vi "PH_Sound.ProcCases.vi"(0 "i ref in":refnum<vi>, 1 "selector":string, 2 "Data":T1, 3 "call cluster":T2={"Object"="", "Selector"="", "CallType"=enum."synchronous", "Async Object"="", "Async Selector"="", "Data Descriptor"="", "Data"=[], "Error #"=0, "Expire"=0}, 5 "error in (no error)":errorcluster) -> (14 "i ref out":refnum<vi>, 17 "answer cluster":T2={"Object"="", "Selector"="", "CallType"=enum."synchronous", "Async Object"="", "Async Selector"="", "Data Descriptor"="", "Data"=[], "Error #"=0, "Expire"=0}, 19 "error out":errorcluster)   [LabVIEW 2014, in "PH_Sound.lvlib"]
doc: "This method is called by a process from within the default case in the event loop. The methods of a class that are linked to events will be called from THIS method. Add your code here."
uses:
  PH_Sound.lvlib
  CS_Core/CSSystem/CoreDefs/CoreDefs.call_type.ctl
  CS_Core/BaseProcess/BaseProcess.descriptor string definition.ctl
  CS_Core/CSSystem/CoreDefs/CoreDefs.rawDataType.ctl
  CS_Core/CSSystem/CoreLib/CoreLib.byte array 2 double.vi
  CS_Core/CSSystem/CoreLib/CoreLib.byte array 2 int.vi
  CS_Core/CSSystem/CoreLib/CoreLib.string 2 byte array.vi
  CS_Core/CSSystem/CoreLib/CoreLib.byte array 2 short.vi
  CS_Core/BaseProcess/BaseProcess.lvlib
  CS_Core/CSSystem/CoreLib/CoreLib.lvlib
  CS_Core/CAEObj/CAEObj.lvlib
  PH_Basics/PH_Common/PH_Common.lvlib
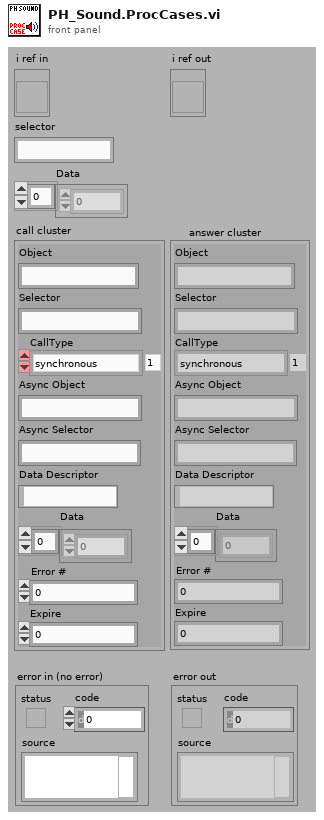
[diagram p1: front panel]
types:
  T1 = typedef "CoreDefs.rawDataType.ctl" = i8[]
  T2 = typedef "CoreDefs.call_type.ctl" = cluster{"Object":string, "Selector":string, "CallType":enum16{"simple", "synchronous", "asynchronous"}, "Async Object":string, "Async Selector":string, "Data Descriptor":T3, "Data":T1, "Error #":i32, "Expire":u32}
  T3 = typedef "BaseProcess.lvlib/BaseProcess.descriptor string definition.ctl" = string
  T4 = typedef "PH_Sound.lvlib/PH_Sound.i attribute.ctl" = cluster{"GUI Refs":cluster{"Exit":refnum<vi>, "Laserfreigabe":refnum<vi>, "PreAmp-Freigabe":refnum<vi>, "Countdown Running":refnum<vi>, "Emergency Off":refnum<vi>, "Device Error":refnum<vi>}, "Testalarm on":bool, "State":cluster{"Laser Class 4":bool, "PreAmp Running":bool, "Countdown Running":bool, "Emergency Off":bool}, "Starting Time":timestamp}
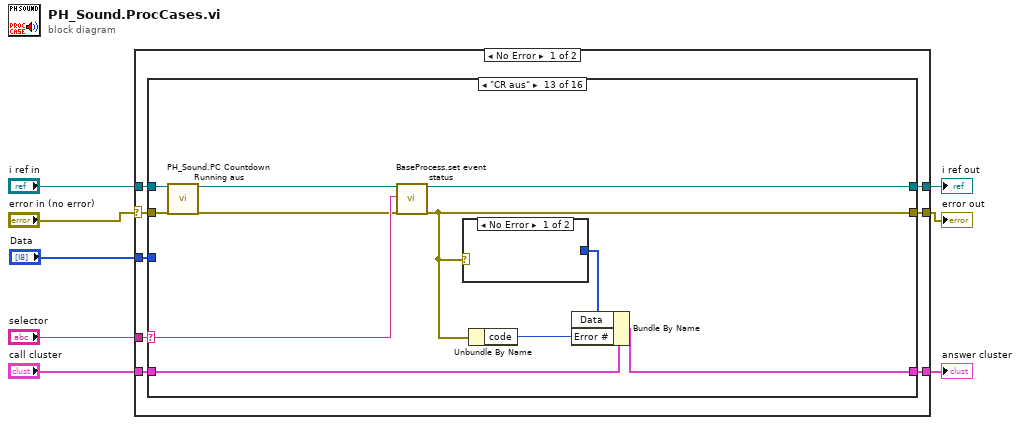
[diagram p0: block diagram]
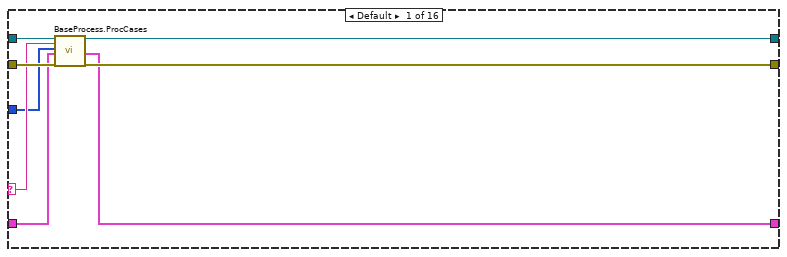
[diagram p2: hidden frame]
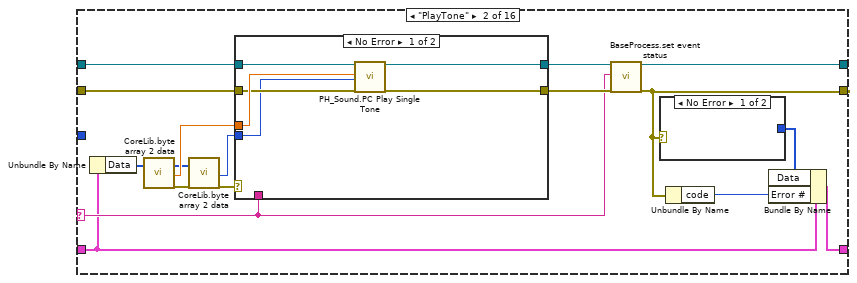
[diagram p3: hidden frame]
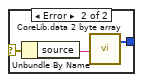
[diagram p4: hidden frame]
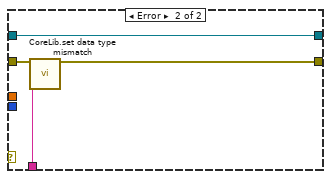
[diagram p5: hidden frame]
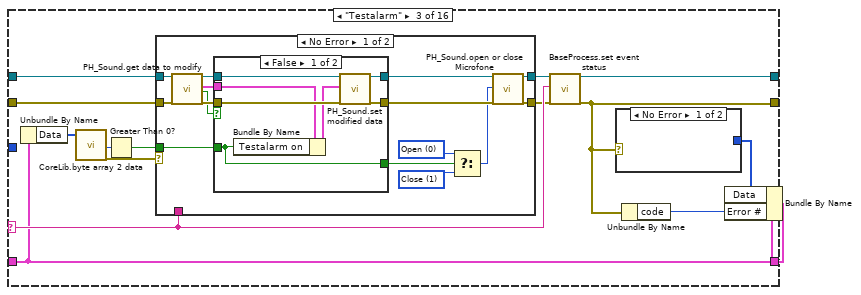
[diagram p6: hidden frame]
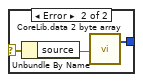
[diagram p7: hidden frame]
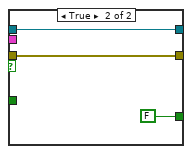
[diagram p8: hidden frame]
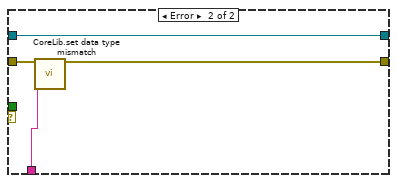
[diagram p9: hidden frame]
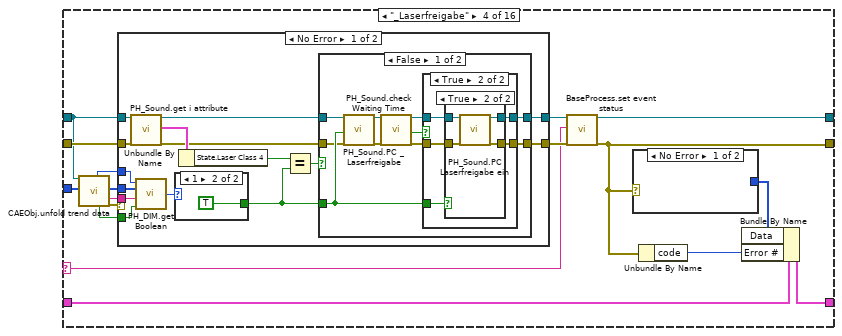
[diagram p10: hidden frame]
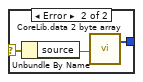
[diagram p11: hidden frame]
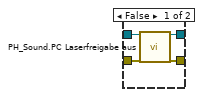
[diagram p13: hidden frame]
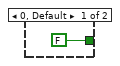
[diagram p15: hidden frame]
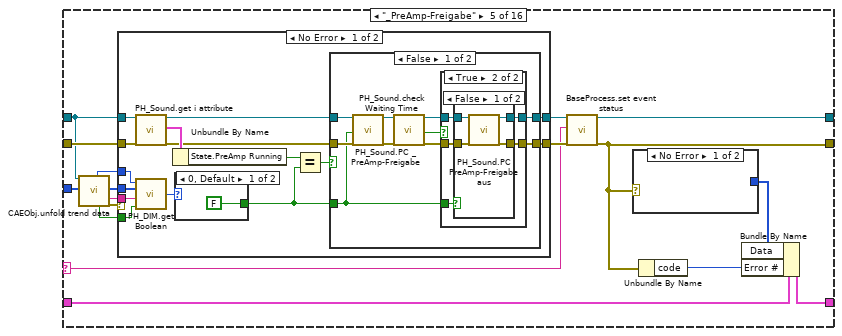
[diagram p17: hidden frame]
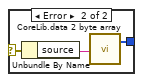
[diagram p18: hidden frame]
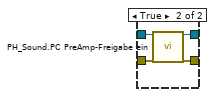
[diagram p20: hidden frame]
diagram:
  n1 = case shown="No Error" "error in (no error)" {
    selector: "error in (no error)" -> [w9 w466]
    tunnel: "selector" -> [w16 _]
    tunnel: [w15 w465] -> w7
    tunnel: "call cluster" -> [w14 w465]
    tunnel: "i ref in" -> [w13 w467]
    tunnel: [w12 w467] -> w4
    tunnel: [w11 w466] -> w3
    tunnel: "Data" -> [w10 _]
    frame No Error {
      n2 = case shown="\"CR aus\"" w16 {
        selector: w16 -> [w19 w31 w61 w105 w171 w237 w304 w341 w353 w367 w381 w395 w413 w427 w441 w455]
        tunnel: w13 -> [w18 w41 w69 w102 w168 w234 w313 w348 w363 w377 w391 w405 w412 w426 w440 w454]
        tunnel: [w24 w33 w58 w107 w173 w239 w301 w343 w357 w371 w385 w399 w417 w431 w445 w459] -> w12
        tunnel: w14 -> [w20 w30 w56 w104 w170 w236 w303 w340 w355 w369 w383 w397 w415 w429 w443 w457]
        tunnel: [w21 w29 w55 w103 w169 w235 w302 w339 w354 w368 w382 w396 w414 w428 w442 w456] -> w15
        tunnel: w9 -> [w23 w40 w68 w118 w184 w250 w316 w349 w362 w376 w390 w404 w411 w425 w439 w453]
        tunnel: [w22 w32 w57 w106 w172 w238 w300 w342 w356 w370 w384 w398 w416 w430 w444 w458] -> w11
        tunnel: w10 -> [w17 _ _ w117 w183 w249 w315 _ _ _ _ _ _ _ _ _]
        frame Default {
          n3 = call "BaseProcess.ProcCases.vi"("i ref in"=w18, "selector"=w19, "Data"=w17, "call cluster"=w20, "error in (no error)"=w23) -> ("i ref out"=w24:refnum<vi>, "answer cluster"=w21:T2, "error out"=w22:errorcluster)  [unwired: 12 in]
        }
        frame "PlayTone" {
          n4 = Unbundle By Name(w30) -> ("Data"=w39:T1)
          n5 = call-poly "CoreLib.byte array 2 data.vi"("byteArray"=w39) -> ("byteArray out"=w26:T1, "d64"=w38:dbl, "error out"=w28:errorcluster)  [unwired: 16 in]
          n6 = call-poly "CoreLib.byte array 2 data.vi"("byteArray"=w26, "error in (no error)"=w28) -> ("i32"=w25:i32, "error out"=w27:errorcluster)  [unwired: 15 in, 1 out]
          n7 = case shown="No Error" w27 {
            tunnel: [w46 w54] -> w35
            tunnel: w41 -> [w49 w54]
            tunnel: w40 -> [w48 w53]
            tunnel: [w47 w52] -> w34
            tunnel: w31 -> [_ w51]
            tunnel: w38 -> [w50 _]
            tunnel: w25 -> [w45 _]
            frame No Error {
              n8 = call "PH_Sound.PC Play Single Tone.vi"("VI in"=w49, "Tone"=w50, "Length [ms]"=w45, "error in (no error)"=w48) -> ("VI out"=w46:refnum<vi>, "error out"=w47:errorcluster)  [unwired: 14 in]
            }
            frame Error {
              n9 = call "CoreLib.set data type mismatch.vi"("error in (no error)"=w53, "error source"=w51) -> ("error out"=w52:errorcluster)  [unwired: 17 in]
            }
          }
          n10 = call "BaseProcess.set event status.vi"("i ref in"=w35, "EventStatus"=w31, "error in (no error)"=w34) -> ("i ref out"=w33:refnum<vi>, "error out"=w32:errorcluster)  [unwired: 14 in, 1 out]
          n11 = case shown="No Error" w32 {
            selector: w32 -> [_ w44]
            tunnel: [_ w42] -> w37
            frame No Error {
            }
            frame Error {
              n12 = Unbundle By Name(w44) -> ("source"=w43:string)
              n13 = call-poly "CoreLib.data 2 byte array.vi"("string"=w43) -> ("byteArray out"=w42:T1)  [unwired: 18 in]
            }
          }
          n14 = Unbundle By Name(w32) -> ("code"=w36:i32)
          n15 = Bundle By Name(cluster=w30, "Data"=w37, "Error #"=w36) -> (w29:T2)
        }
        frame "Testalarm" {
          n16 = Unbundle By Name(w56) -> ("Data"=w66:T1)
          n17 = call-poly "CoreLib.byte array 2 data.vi"("byteArray"=w66) -> ("i16"=w67:i16, "error out"=w65:errorcluster)  [unwired: 16 in, 1 out]
          n18 = Greater Than 0?(x=w67) -> (x > 0?=w64:bool)
          n19 = case shown="No Error" w65 {
            tunnel: [w78 w101] -> w59
            tunnel: w69 -> [w87 w101]
            tunnel: w68 -> [w86 w100]
            tunnel: [w76 w99] -> w60
            tunnel: w61 -> [_ w98]
            tunnel: w64 -> [w82 _]
            frame No Error {
              w79 = u16 1 items=["Open", "Close"] ("Action")
              w80 = u16 0 items=["Open", "Close"] ("Action")
              n20 = call "PH_Sound.get data to modify.vi"("i ref in"=w87, "error in (no error)"=w86) -> ("i ref out"=w84:refnum<vi>, "i attribute"=w83:T4, "timed out"=w81:bool, "error out"=w85:errorcluster)  [unwired: 14 in]
              n21 = case shown="False" w81 {
                tunnel: w85 -> [w94 w96]
                tunnel: w84 -> [w93 w97]
                tunnel: [w92 w97] -> w77
                tunnel: [w91 w96] -> w75
                tunnel: w83 -> [w90 _]
                tunnel: w82 -> [w88 _]
                tunnel: [w88 FALSE ("err")] -> w74
                frame False {
                  n22 = Bundle By Name(cluster=w90, "Testalarm on"=w88) -> (w89:T4)
                  n23 = call "PH_Sound.set modified data.vi"("i ref in"=w93, "i attribute"=w89, "error in (no error)"=w94) -> ("i ref out"=w92:refnum<vi>, "error out"=w91:errorcluster)  [unwired: 15 in]
                }
                frame True {
                }
              }
              n24 = Select(t=w80, s=w74, f=w79) -> (s? t:f=w73:u16)
              n25 = call "PH_Sound.open or close Microfone.vi"("i ref in"=w77, "Action"=w73, "error in (no error)"=w75) -> ("i ref out"=w78:refnum<vi>, "error out"=w76:errorcluster)  [unwired: 15 in]
            }
            frame Error {
              n26 = call "CoreLib.set data type mismatch.vi"("error in (no error)"=w100, "error source"=w98) -> ("error out"=w99:errorcluster)  [unwired: 17 in]
            }
          }
          n27 = call "BaseProcess.set event status.vi"("i ref in"=w59, "EventStatus"=w61, "error in (no error)"=w60) -> ("i ref out"=w58:refnum<vi>, "error out"=w57:errorcluster)  [unwired: 14 in, 1 out]
          n28 = case shown="No Error" w57 {
            selector: w57 -> [_ w72]
            tunnel: [_ w70] -> w63
            frame No Error {
            }
            frame Error {
              n29 = Unbundle By Name(w72) -> ("source"=w71:string)
              n30 = call-poly "CoreLib.data 2 byte array.vi"("string"=w71) -> ("byteArray out"=w70:T1)  [unwired: 18 in]
            }
          }
          n31 = Unbundle By Name(w57) -> ("code"=w62:i32)
          n32 = Bundle By Name(cluster=w56, "Data"=w63, "Error #"=w62) -> (w55:T2)
        }
        frame "_Laserfreigabe" {
          n33 = call "CAEObj.unfold trend data.vi"("i ref in"=w102, "raw trend data"=w117) -> ("quality"=w112:i32, "no link"=w113:bool, "data"=w114:i8[], "typeDescriptor"=w115:string, "error out"=w116:errorcluster)  [unwired: 9 in, 4 out]
          n34 = case shown="No Error" w116 {
            tunnel: [w132 w167] -> w108
            tunnel: w102 -> [w136 w167]
            tunnel: w118 -> [w135 w166]
            tunnel: [w131 w166] -> w109
            tunnel: w115 -> [w130 _]
            tunnel: w114 -> [w129 _]
            tunnel: w113 -> [w128 _]
            tunnel: w112 -> [w127 _]
            frame No Error {
              n35 = call "PH_Sound.get i attribute.vi"("i ref in"=w136, "error in (no error)"=w135) -> ("i ref out"=w123:refnum<vi>, "i attribute"=w134:T4, "error out"=w122:errorcluster)  [unwired: 15 in]
              n36 = call "PH_DIM.get Boolean.vi"("no link"=w128, "typeDescriptor"=w130, "data"=w129, "quality"=w127) -> ("Value"=w126:i32)
              n37 = case shown="1" w126 {
                tunnel: [FALSE TRUE] -> w125
                frame 0, Default {
                }
                frame 1 {
                }
              }
              n38 = Unbundle By Name(w134) -> ("State.Laser Class 4"=w133:bool)
              n39 = Equal?(x=w133, y=w125) -> (x = y?=w124:bool)
              n40 = case shown="False" w124 {
                tunnel: w123 -> [w143 w163]
                tunnel: [w146 w163] -> w132
                tunnel: w122 -> [w142 w162]
                tunnel: [w145 w162] -> w131
                tunnel: w125 -> [w144 _]
                frame False {
                  n41 = call "PH_Sound.PC _Laserfreigabe.vi"("i ref in"=w143, "State Laserfreigabe"=w144, "error in (no error)"=w142) -> ("i ref out"=w141:refnum<vi>, "error out"=w139:errorcluster)  [unwired: 15 in]
                  n42 = call "PH_Sound.check Waiting Time.vi"("i ref in"=w141, "error in"=w139) -> ("i ref out"=w140:refnum<vi>, "Waiting Time over?"=w137:bool, "error out"=w138:errorcluster)  [unwired: 15 in]
                  n43 = case shown="True" w137 {
                    tunnel: [w148 w153] -> w146
                    tunnel: [w147 w152] -> w145
                    tunnel: w144 -> [_ w151]
                    tunnel: w140 -> [w148 w150]
                    tunnel: w138 -> [w147 w149]
                    frame False {
                    }
                    frame True {
                      n44 = case shown="True" w151 {
                        tunnel: w150 -> [w155 w159]
                        tunnel: [w154 w158] -> w153
                        tunnel: w149 -> [w157 w161]
                        tunnel: [w156 w160] -> w152
                        frame False {
                          n45 = call "PH_Sound.PC Laserfreigabe aus.vi"("i ref in"=w155, "error IO"=w157) -> ("i ref out"=w154:refnum<vi>, "error out"=w156:errorcluster)  [unwired: 16 in]
                        }
                        frame True {
                          n46 = call "PH_Sound.PC Laserfreigabe ein.vi"("i ref in"=w159, "error IO"=w161) -> ("i ref out"=w158:refnum<vi>, "error out"=w160:errorcluster)  [unwired: 16 in]
                        }
                      }
                    }
                  }
                }
                frame True {
                }
              }
            }
            frame Error {
            }
          }
          n47 = call "BaseProcess.set event status.vi"("i ref in"=w108, "EventStatus"=w105, "error in (no error)"=w109) -> ("i ref out"=w107:refnum<vi>, "error out"=w106:errorcluster)  [unwired: 14 in, 1 out]
          n48 = case shown="No Error" w106 {
            selector: w106 -> [_ w121]
            tunnel: [_ w119] -> w111
            frame No Error {
            }
            frame Error {
              n49 = Unbundle By Name(w121) -> ("source"=w120:string)
              n50 = call-poly "CoreLib.data 2 byte array.vi"("string"=w120) -> ("byteArray out"=w119:T1)  [unwired: 18 in]
            }
          }
          n51 = Unbundle By Name(w106) -> ("code"=w110:i32)
          n52 = Bundle By Name(cluster=w104, "Data"=w111, "Error #"=w110) -> (w103:T2)
        }
        frame "_PreAmp-Freigabe" {
          n53 = call "CAEObj.unfold trend data.vi"("i ref in"=w168, "raw trend data"=w183) -> ("quality"=w178:i32, "no link"=w179:bool, "data"=w180:i8[], "typeDescriptor"=w181:string, "error out"=w182:errorcluster)  [unwired: 9 in, 4 out]
          n54 = case shown="No Error" w182 {
            tunnel: [w198 w233] -> w174
            tunnel: w168 -> [w202 w233]
            tunnel: w184 -> [w201 w232]
            tunnel: [w197 w232] -> w175
            tunnel: w181 -> [w196 _]
            tunnel: w180 -> [w195 _]
            tunnel: w179 -> [w194 _]
            tunnel: w178 -> [w193 _]
            frame No Error {
              n55 = call "PH_Sound.get i attribute.vi"("i ref in"=w202, "error in (no error)"=w201) -> ("i ref out"=w189:refnum<vi>, "i attribute"=w200:T4, "error out"=w188:errorcluster)  [unwired: 15 in]
              n56 = call "PH_DIM.get Boolean.vi"("no link"=w194, "typeDescriptor"=w196, "data"=w195, "quality"=w193) -> ("Value"=w192:i32)
              n57 = Unbundle By Name(w200) -> ("State.PreAmp Running"=w199:bool)
              n58 = case shown="0, Default" w192 {
                tunnel: [FALSE TRUE] -> w191
                frame 0, Default {
                }
                frame 1 {
                }
              }
              n59 = Equal?(x=w199, y=w191) -> (x = y?=w190:bool)
              n60 = case shown="False" w190 {
                tunnel: w189 -> [w208 w229]
                tunnel: [w212 w229] -> w198
                tunnel: w188 -> [w207 w228]
                tunnel: [w211 w228] -> w197
                tunnel: w191 -> [w204 _]
                frame False {
                  n61 = call "PH_Sound.PC _PreAmp-Freigabe.vi"("i ref in"=w208, "State PreAmp-Freigabe"=w204, "error in (no error)"=w207) -> ("i ref out"=w209:refnum<vi>, "error out"=w210:errorcluster)  [unwired: 15 in]
                  n62 = call "PH_Sound.check Waiting Time.vi"("i ref in"=w209, "error in"=w210) -> ("i ref out"=w205:refnum<vi>, "Waiting Time over?"=w203:bool, "error out"=w206:errorcluster)  [unwired: 15 in]
                  n63 = case shown="True" w203 {
                    tunnel: [w214 w219] -> w212
                    tunnel: [w213 w218] -> w211
                    tunnel: w206 -> [w213 w217]
                    tunnel: w205 -> [w214 w216]
                    tunnel: w204 -> [_ w215]
                    frame False {
                    }
                    frame True {
                      n64 = case shown="False" w215 {
                        tunnel: w216 -> [w221 w225]
                        tunnel: [w220 w224] -> w219
                        tunnel: w217 -> [w223 w227]
                        tunnel: [w222 w226] -> w218
                        frame False {
                          n65 = call "PH_Sound.PC PreAmp-Freigabe aus.vi"("i ref in"=w221, "error IO"=w223) -> ("i ref out"=w220:refnum<vi>, "error out"=w222:errorcluster)  [unwired: 16 in]
                        }
                        frame True {
                          n66 = call "PH_Sound.PC PreAmp-Freigabe ein.vi"("i ref in"=w225, "error IO"=w227) -> ("i ref out"=w224:refnum<vi>, "error out"=w226:errorcluster)  [unwired: 16 in]
                        }
                      }
                    }
                  }
                }
                frame True {
                }
              }
            }
            frame Error {
            }
          }
          n67 = call "BaseProcess.set event status.vi"("i ref in"=w174, "EventStatus"=w171, "error in (no error)"=w175) -> ("i ref out"=w173:refnum<vi>, "error out"=w172:errorcluster)  [unwired: 14 in, 1 out]
          n68 = case shown="No Error" w172 {
            selector: w172 -> [_ w187]
            tunnel: [_ w185] -> w177
            frame No Error {
            }
            frame Error {
              n69 = Unbundle By Name(w187) -> ("source"=w186:string)
              n70 = call-poly "CoreLib.data 2 byte array.vi"("string"=w186) -> ("byteArray out"=w185:T1)  [unwired: 18 in]
            }
          }
          n71 = Unbundle By Name(w172) -> ("code"=w176:i32)
          n72 = Bundle By Name(cluster=w170, "Data"=w177, "Error #"=w176) -> (w169:T2)
        }
        frame "_CountdownRunning" {
          n73 = call "CAEObj.unfold trend data.vi"("i ref in"=w234, "raw trend data"=w249) -> ("quality"=w244:i32, "no link"=w245:bool, "data"=w246:i8[], "typeDescriptor"=w247:string, "error out"=w248:errorcluster)  [unwired: 9 in, 4 out]
          n74 = case shown="No Error" w248 {
            tunnel: [w264 w299] -> w240
            tunnel: w234 -> [w268 w299]
            tunnel: w250 -> [w267 w298]
            tunnel: [w263 w298] -> w241
            tunnel: w247 -> [w262 _]
            tunnel: w246 -> [w261 _]
            tunnel: w245 -> [w260 _]
            tunnel: w244 -> [w259 _]
            frame No Error {
              n75 = call "PH_Sound.get i attribute.vi"("i ref in"=w268, "error in (no error)"=w267) -> ("i ref out"=w256:refnum<vi>, "i attribute"=w266:T4, "error out"=w255:errorcluster)  [unwired: 15 in]
              n76 = call "PH_DIM.get Boolean.vi"("no link"=w260, "typeDescriptor"=w262, "data"=w261, "quality"=w259) -> ("Value"=w258:i32)
              n77 = Unbundle By Name(w266) -> ("State.Countdown Running"=w265:bool)
              n78 = case shown="2" w258 {
                tunnel: [FALSE TRUE] -> w257
                frame 0, Default {
                }
                frame 2 {
                }
              }
              n79 = Equal?(x=w265, y=w257) -> (x = y?=w254:bool)
              n80 = case shown="False" w254 {
                tunnel: w256 -> [w274 w295]
                tunnel: [w278 w295] -> w264
                tunnel: w255 -> [w272 w294]
                tunnel: [w277 w294] -> w263
                tunnel: w257 -> [w270 _]
                frame False {
                  n81 = call "PH_Sound.PC _CountdownRunning.vi"("i ref in"=w274, "State CR"=w270, "error in (no error)"=w272) -> ("i ref out"=w275:refnum<vi>, "error out"=w276:errorcluster)  [unwired: 15 in]
                  n82 = call "PH_Sound.check Waiting Time.vi"("i ref in"=w275, "error in"=w276) -> ("i ref out"=w273:refnum<vi>, "Waiting Time over?"=w269:bool, "error out"=w271:errorcluster)  [unwired: 15 in]
                  n83 = case shown="True" w269 {
                    tunnel: [w280 w285] -> w278
                    tunnel: [w279 w284] -> w277
                    tunnel: w273 -> [w280 w283]
                    tunnel: w271 -> [w279 w282]
                    tunnel: w270 -> [_ w281]
                    frame False {
                    }
                    frame True {
                      n84 = case shown="True" w281 {
                        tunnel: w283 -> [w289 w293]
                        tunnel: [w286 w292] -> w285
                        tunnel: w282 -> [w288 w291]
                        tunnel: [w287 w290] -> w284
                        frame False {
                          n85 = call "PH_Sound.PC Countdown Running aus.vi"("i ref in"=w289, "error IO"=w288) -> ("i ref out"=w286:refnum<vi>, "error out"=w287:errorcluster)  [unwired: 16 in]
                        }
                        frame True {
                          n86 = call "PH_Sound.PC Countdown Running ein.vi"("i ref in"=w293, "error IO"=w291) -> ("i ref out"=w292:refnum<vi>, "error out"=w290:errorcluster)  [unwired: 16 in]
                        }
                      }
                    }
                  }
                }
                frame True {
                }
              }
            }
            frame Error {
            }
          }
          n87 = call "BaseProcess.set event status.vi"("i ref in"=w240, "EventStatus"=w237, "error in (no error)"=w241) -> ("i ref out"=w239:refnum<vi>, "error out"=w238:errorcluster)  [unwired: 14 in, 1 out]
          n88 = case shown="Error" w238 {
            selector: w238 -> [_ w253]
            tunnel: [_ w251] -> w243
            frame No Error {
            }
            frame Error {
              n89 = Unbundle By Name(w253) -> ("source"=w252:string)
              n90 = call-poly "CoreLib.data 2 byte array.vi"("string"=w252) -> ("byteArray out"=w251:T1)  [unwired: 18 in]
            }
          }
          n91 = Unbundle By Name(w238) -> ("code"=w242:i32)
          n92 = Bundle By Name(cluster=w236, "Data"=w243, "Error #"=w242) -> (w235:T2)
        }
        frame "_EmergencyOff" {
          n93 = call "CAEObj.unfold trend data.vi"("i ref in"=w313, "raw trend data"=w315) -> ("quality"=w312:i32, "no link"=w309:bool, "data"=w311:i8[], "typeDescriptor"=w310:string, "error out"=w314:errorcluster)  [unwired: 9 in, 4 out]
          n94 = case shown="No Error" w314 {
            tunnel: [w331 w338] -> w305
            tunnel: w313 -> [w334 w338]
            tunnel: w316 -> [w333 w337]
            tunnel: [w329 w337] -> w306
            tunnel: w312 -> [w324 _]
            tunnel: w311 -> [w323 _]
            tunnel: w310 -> [w322 _]
            tunnel: w309 -> [w321 _]
            frame No Error {
              w326 = u16 1 items=["Open", "Close"] ("Action")
              w328 = u16 0 items=["Open", "Close"] ("Action")
              n95 = call "PH_DIM.get Boolean.vi"("no link"=w321, "typeDescriptor"=w322, "data"=w323, "quality"=w324) -> ("Value"=w325:i32)
              n96 = case shown="0, Default" w325 {
                tunnel: [FALSE TRUE] -> w320
                frame 0, Default {
                }
                frame 2 {
                }
              }
              n97 = call "PH_Sound.PC _EmergencyOff.vi"("i ref in"=w334, "State Emernegncy Off"=w320, "error in (no error)"=w333) -> ("i ref out"=w332:refnum<vi>, "error out"=w330:errorcluster)  [unwired: 15 in]
              n98 = Select(t=w328, s=w320, f=w326) -> (s? t:f=w327:u16)
              n99 = call "PH_Sound.open or close Microfone.vi"("i ref in"=w332, "Action"=w327, "error in (no error)"=w330) -> ("i ref out"=w331:refnum<vi>, "error out"=w329:errorcluster)  [unwired: 15 in]
            }
            frame Error {
            }
          }
          n100 = call "BaseProcess.set event status.vi"("i ref in"=w305, "EventStatus"=w304, "error in (no error)"=w306) -> ("i ref out"=w301:refnum<vi>, "error out"=w300:errorcluster)  [unwired: 14 in, 1 out]
          n101 = case shown="No Error" w300 {
            selector: w300 -> [_ w319]
            tunnel: [_ w317] -> w308
            frame No Error {
            }
            frame Error {
              n102 = Unbundle By Name(w319) -> ("source"=w318:string)
              n103 = call-poly "CoreLib.data 2 byte array.vi"("string"=w318) -> ("byteArray out"=w317:T1)  [unwired: 18 in]
            }
          }
          n104 = Unbundle By Name(w300) -> ("code"=w307:i32)
          n105 = Bundle By Name(cluster=w303, "Data"=w308, "Error #"=w307) -> (w302:T2)
        }
        frame "Laserfreigabe ein" {
          n106 = call "PH_Sound.PC Laserfreigabe ein.vi"("i ref in"=w348, "error IO"=w349) -> ("i ref out"=w344:refnum<vi>, "error out"=w345:errorcluster)  [unwired: 16 in]
          n107 = call "BaseProcess.set event status.vi"("i ref in"=w344, "EventStatus"=w341, "error in (no error)"=w345) -> ("i ref out"=w343:refnum<vi>, "error out"=w342:errorcluster)  [unwired: 14 in, 1 out]
          n108 = case shown="No Error" w342 {
            selector: w342 -> [_ w352]
            tunnel: [_ w350] -> w347
            frame No Error {
            }
            frame Error {
              n109 = Unbundle By Name(w352) -> ("source"=w351:string)
              n110 = call-poly "CoreLib.data 2 byte array.vi"("string"=w351) -> ("byteArray out"=w350:T1)  [unwired: 18 in]
            }
          }
          n111 = Unbundle By Name(w342) -> ("code"=w346:i32)
          n112 = Bundle By Name(cluster=w340, "Data"=w347, "Error #"=w346) -> (w339:T2)
        }
        frame "Laserfreigabe aus" {
          n113 = call "PH_Sound.PC Laserfreigabe aus.vi"("i ref in"=w363, "error IO"=w362) -> ("i ref out"=w358:refnum<vi>, "error out"=w359:errorcluster)  [unwired: 16 in]
          n114 = call "BaseProcess.set event status.vi"("i ref in"=w358, "EventStatus"=w353, "error in (no error)"=w359) -> ("i ref out"=w357:refnum<vi>, "error out"=w356:errorcluster)  [unwired: 14 in, 1 out]
          n115 = case shown="No Error" w356 {
            selector: w356 -> [_ w366]
            tunnel: [_ w364] -> w361
            frame No Error {
            }
            frame Error {
              n116 = Unbundle By Name(w366) -> ("source"=w365:string)
              n117 = call-poly "CoreLib.data 2 byte array.vi"("string"=w365) -> ("byteArray out"=w364:T1)  [unwired: 18 in]
            }
          }
          n118 = Unbundle By Name(w356) -> ("code"=w360:i32)
          n119 = Bundle By Name(cluster=w355, "Data"=w361, "Error #"=w360) -> (w354:T2)
        }
        frame "PA-Freigabe ein" {
          n120 = call "PH_Sound.PC PreAmp-Freigabe ein.vi"("i ref in"=w377, "error IO"=w376) -> ("i ref out"=w372:refnum<vi>, "error out"=w373:errorcluster)  [unwired: 16 in]
          n121 = call "BaseProcess.set event status.vi"("i ref in"=w372, "EventStatus"=w367, "error in (no error)"=w373) -> ("i ref out"=w371:refnum<vi>, "error out"=w370:errorcluster)  [unwired: 14 in, 1 out]
          n122 = case shown="No Error" w370 {
            selector: w370 -> [_ w380]
            tunnel: [_ w378] -> w375
            frame No Error {
            }
            frame Error {
              n123 = Unbundle By Name(w380) -> ("source"=w379:string)
              n124 = call-poly "CoreLib.data 2 byte array.vi"("string"=w379) -> ("byteArray out"=w378:T1)  [unwired: 18 in]
            }
          }
          n125 = Unbundle By Name(w370) -> ("code"=w374:i32)
          n126 = Bundle By Name(cluster=w369, "Data"=w375, "Error #"=w374) -> (w368:T2)
        }
        frame "PA-Freigabe aus" {
          n127 = call "PH_Sound.PC PreAmp-Freigabe aus.vi"("i ref in"=w391, "error IO"=w390) -> ("i ref out"=w386:refnum<vi>, "error out"=w387:errorcluster)  [unwired: 16 in]
          n128 = call "BaseProcess.set event status.vi"("i ref in"=w386, "EventStatus"=w381, "error in (no error)"=w387) -> ("i ref out"=w385:refnum<vi>, "error out"=w384:errorcluster)  [unwired: 14 in, 1 out]
          n129 = case shown="No Error" w384 {
            selector: w384 -> [_ w394]
            tunnel: [_ w392] -> w389
            frame No Error {
            }
            frame Error {
              n130 = Unbundle By Name(w394) -> ("source"=w393:string)
              n131 = call-poly "CoreLib.data 2 byte array.vi"("string"=w393) -> ("byteArray out"=w392:T1)  [unwired: 18 in]
            }
          }
          n132 = Unbundle By Name(w384) -> ("code"=w388:i32)
          n133 = Bundle By Name(cluster=w383, "Data"=w389, "Error #"=w388) -> (w382:T2)
        }
        frame "CR ein" {
          n134 = call "PH_Sound.PC Countdown Running ein.vi"("i ref in"=w405, "error IO"=w404) -> ("i ref out"=w400:refnum<vi>, "error out"=w401:errorcluster)  [unwired: 16 in]
          n135 = call "BaseProcess.set event status.vi"("i ref in"=w400, "EventStatus"=w395, "error in (no error)"=w401) -> ("i ref out"=w399:refnum<vi>, "error out"=w398:errorcluster)  [unwired: 14 in, 1 out]
          n136 = case shown="No Error" w398 {
            selector: w398 -> [_ w408]
            tunnel: [_ w406] -> w403
            frame No Error {
            }
            frame Error {
              n137 = Unbundle By Name(w408) -> ("source"=w407:string)
              n138 = call-poly "CoreLib.data 2 byte array.vi"("string"=w407) -> ("byteArray out"=w406:T1)  [unwired: 18 in]
            }
          }
          n139 = Unbundle By Name(w398) -> ("code"=w402:i32)
          n140 = Bundle By Name(cluster=w397, "Data"=w403, "Error #"=w402) -> (w396:T2)
        }
        frame "CR aus" {
          n141 = call "PH_Sound.PC Countdown Running aus.vi"("i ref in"=w412, "error IO"=w411) -> ("i ref out"=w410:refnum<vi>, "error out"=w409:errorcluster)  [unwired: 16 in]
          n142 = call "BaseProcess.set event status.vi"("i ref in"=w410, "EventStatus"=w413, "error in (no error)"=w409) -> ("i ref out"=w417:refnum<vi>, "error out"=w416:errorcluster)  [unwired: 14 in, 1 out]
          n143 = case shown="No Error" w416 {
            selector: w416 -> [_ w422]
            tunnel: [_ w420] -> w419
            frame No Error {
            }
            frame Error {
              n144 = Unbundle By Name(w422) -> ("source"=w421:string)
              n145 = call-poly "CoreLib.data 2 byte array.vi"("string"=w421) -> ("byteArray out"=w420:T1)  [unwired: 18 in]
            }
          }
          n146 = Unbundle By Name(w416) -> ("code"=w418:i32)
          n147 = Bundle By Name(cluster=w415, "Data"=w419, "Error #"=w418) -> (w414:T2)
        }
        frame "Timing 1" {
          n148 = call "PH_Sound.PC Timing 1.vi"("i ref in"=w426, "error IO"=w425) -> ("i ref out"=w424:refnum<vi>, "error out"=w423:errorcluster)  [unwired: 16 in]
          n149 = call "BaseProcess.set event status.vi"("i ref in"=w424, "EventStatus"=w427, "error in (no error)"=w423) -> ("i ref out"=w431:refnum<vi>, "error out"=w430:errorcluster)  [unwired: 14 in, 1 out]
          n150 = case shown="No Error" w430 {
            selector: w430 -> [_ w436]
            tunnel: [_ w434] -> w433
            frame No Error {
            }
            frame Error {
              n151 = Unbundle By Name(w436) -> ("source"=w435:string)
              n152 = call-poly "CoreLib.data 2 byte array.vi"("string"=w435) -> ("byteArray out"=w434:T1)  [unwired: 18 in]
            }
          }
          n153 = Unbundle By Name(w430) -> ("code"=w432:i32)
          n154 = Bundle By Name(cluster=w429, "Data"=w433, "Error #"=w432) -> (w428:T2)
        }
        frame "Timing 2" {
          n155 = call "PH_Sound.PC Timing 2.vi"("i ref in"=w440, "error IO"=w439) -> ("i ref out"=w438:refnum<vi>, "error out"=w437:errorcluster)  [unwired: 16 in]
          n156 = call "BaseProcess.set event status.vi"("i ref in"=w438, "EventStatus"=w441, "error in (no error)"=w437) -> ("i ref out"=w445:refnum<vi>, "error out"=w444:errorcluster)  [unwired: 14 in, 1 out]
          n157 = case shown="No Error" w444 {
            selector: w444 -> [_ w450]
            tunnel: [_ w448] -> w447
            frame No Error {
            }
            frame Error {
              n158 = Unbundle By Name(w450) -> ("source"=w449:string)
              n159 = call-poly "CoreLib.data 2 byte array.vi"("string"=w449) -> ("byteArray out"=w448:T1)  [unwired: 18 in]
            }
          }
          n160 = Unbundle By Name(w444) -> ("code"=w446:i32)
          n161 = Bundle By Name(cluster=w443, "Data"=w447, "Error #"=w446) -> (w442:T2)
        }
        frame "Timing 3" {
          n162 = call "PH_Sound.PC Timing 3.vi"("i ref in"=w454, "error IO"=w453) -> ("i ref out"=w452:refnum<vi>, "error out"=w451:errorcluster)  [unwired: 16 in]
          n163 = call "BaseProcess.set event status.vi"("i ref in"=w452, "EventStatus"=w455, "error in (no error)"=w451) -> ("i ref out"=w459:refnum<vi>, "error out"=w458:errorcluster)  [unwired: 14 in, 1 out]
          n164 = case shown="No Error" w458 {
            selector: w458 -> [_ w464]
            tunnel: [_ w462] -> w461
            frame No Error {
            }
            frame Error {
              n165 = Unbundle By Name(w464) -> ("source"=w463:string)
              n166 = call-poly "CoreLib.data 2 byte array.vi"("string"=w463) -> ("byteArray out"=w462:T1)  [unwired: 18 in]
            }
          }
          n167 = Unbundle By Name(w458) -> ("code"=w460:i32)
          n168 = Bundle By Name(cluster=w457, "Data"=w461, "Error #"=w460) -> (w456:T2)
        }
      }
    }
    frame Error {
    }
  }
  "answer cluster" <- w7
  "i ref out" <- w4
  "error out" <- w3
